vi "Apply Force.vi"(8 "error in":errorcluster, 10 "Force Vector":refnum<class "PVector.lvclass">, 11 "Mover in":refnum<class "Mover.lvclass">) -> (0 "error out":errorcluster, 3 "Mover out":refnum<class "Mover.lvclass">)   [LabVIEW 2016, in "Mover.lvclass"]
doc: "Applies Force vector to Mover by adding force components to its Acceleration vector.\nThe force is scaled by inverse of Mover's mass."
uses:
  Mover.lvclass
  PVector/PVector.lvclass
  Mover.lvclass/Mover.ctl
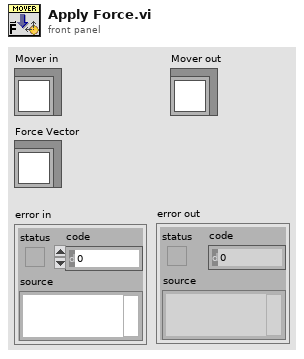
[diagram p1: front panel]
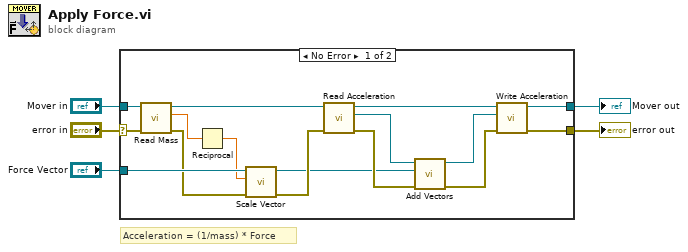
[diagram p0: block diagram]
diagram:
  # "Acceleration = (1/mass) * Force"
  n1 = case shown="No Error" "error in" {
    selector: "error in" -> [w12 w23]
    tunnel: [w15 w23] -> w4
    tunnel: [w16 w22] -> w2
    tunnel: "Mover in" -> [w14 w22]
    tunnel: "Force Vector" -> [w11 _]
    frame No Error {
      n2 = call "Read Mass.vi"("error in"=w12, "Mover in"=w14) -> ("error out"=w8:errorcluster, "Mass"=w10:dbl, "Mover out"=w13:refnum<class "Mover.lvclass">)  [unwired: 7 in]
      n3 = Reciprocal(x=w10) -> (1/x=w9:dbl)
      n4 = call "Scale Vector.vi"("error in"=w8, "n (1)"=w9, "PVector V"=w11) -> ("error out"=w7:errorcluster, "PVector nV"=w6:refnum<class "PVector.lvclass">)  [unwired: 7 in]
      n5 = call "Read Acceleration.vi"("error in"=w7, "Mover in"=w13) -> ("error out"=w20:errorcluster, "Acceleration PVector"=w21:refnum<class "PVector.lvclass">, "Mover out"=w19:refnum<class "Mover.lvclass">)  [unwired: 7 in]
      n6 = call "Add Vectors.vi"("error in"=w20, "PVector U"=w6, "PVector V"=w21) -> ("error out"=w17:errorcluster, "PVector (V+U)"=w18:refnum<class "PVector.lvclass">)  [unwired: 7 in]
      n7 = call "Write Acceleration.vi"("error in"=w17, "Acceleration PVector"=w18, "Mover in"=w19) -> ("error out"=w15:errorcluster, "Mover out"=w16:refnum<class "Mover.lvclass">)  [unwired: 7 in]
    }
    frame Error {
    }
  }
  "error out" <- w4
  "Mover out" <- w2
